vi "3.labtask2 (1).vi"() -> ()   [LabVIEW 2022 SP3]
panel:
  out "Array":dbl[](array[numeric])
  out "Waveform Chart":dynamicdata(graph)
  out "Total execution time (s)":u32
  out "Sampling period (ms)":dbl
  out "Total number of samples":dbl
  in  "Sampling rate (Hz)":dbl
  in  "Total duration (s)":dbl
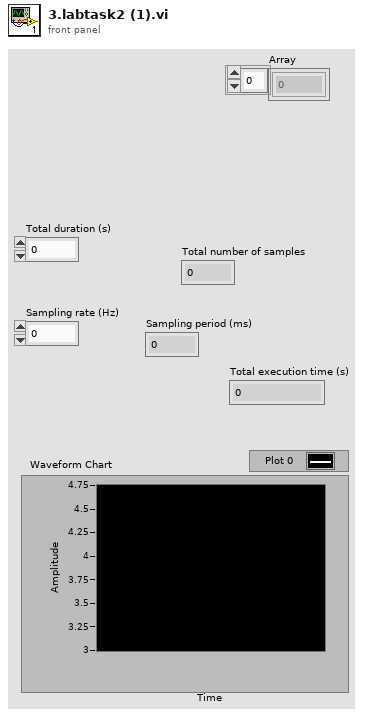
[diagram p1: front panel]
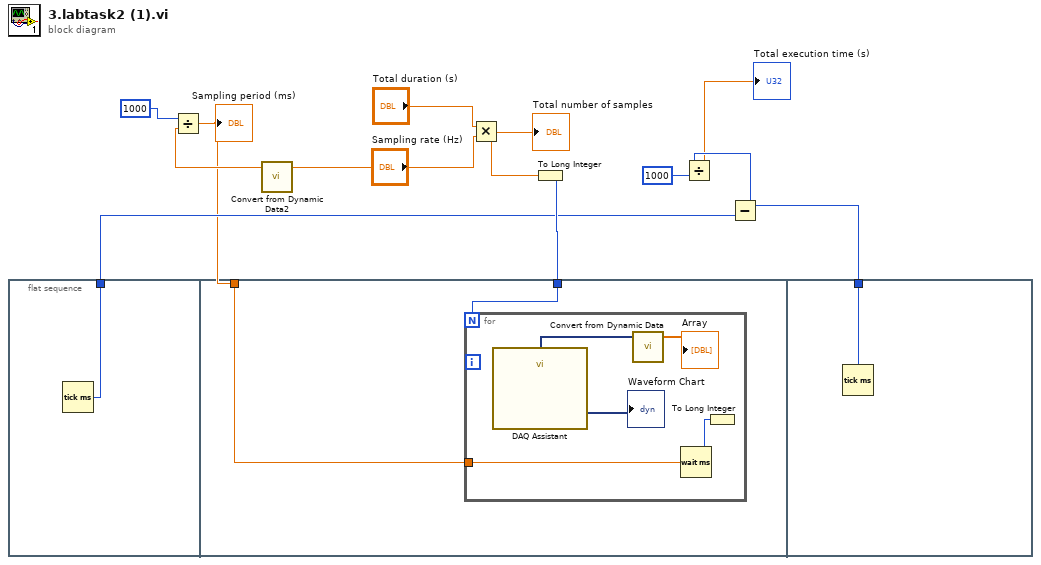
[diagram p0: block diagram]
diagram:
  n1 = flat-sequence {
    tunnel: [w12] -> w2
    tunnel: w7 -> [w14]
    tunnel: w1 -> [w13]
    tunnel: [w19] -> w3
    frame #0 {
      n2 = Tick Count (ms)() -> (millisecond timer value=w12:u32)
    }
    frame #1 {
      n3 = for {
        N: w14 -> [_]
        tunnel: w13 -> [w18]
        n4 = call "DAQ Assistant"() -> ("data"=w16:dynamicdata)  [unwired: 17 in, 2 out]
        "Waveform Chart" <- w16
        n5 = call "Convert from Dynamic Data"("Dynamic Data Type"=w16) -> ("Array"=→"Array":dbl[])  [unwired: 3 in]
        n6 = Wait (ms)(milliseconds to wait=w18) -> (millisecond timer value=w17:u32)
        n7 = To Long Integer(number=w17) -> ()  [unwired: 1 out]
      }
    }
    frame #2 {
      n8 = Tick Count (ms)() -> (millisecond timer value=w19:u32)
    }
  }
  n9 = Divide(x=1000, y="Sampling rate (Hz)") -> (x/y=w1:dbl)
  "Sampling period (ms)" <- w1
  n10 = call "Convert from Dynamic Data2"() -> ()  [unwired: 4 in, 1 out]
  n11 = Multiply(x="Total duration (s)", y="Sampling rate (Hz)") -> (x*y=w11:dbl)
  "Total number of samples" <- w11
  n12 = To Long Integer(number=w11) -> (32bit integer=w7:i32)
  n13 = Subtract(x=w3, y=w2) -> (x-y=w6:u32)
  n14 = Divide(x=w6, y=u32 1000) -> (x/y=→"Total execution time (s)":dbl)
